vi "dv(SubVI).vi"(1 "Array in":dbl[][](array[numeric])) -> (0 "Array":dbl[][][](array[numeric]))   [LabVIEW 2021]
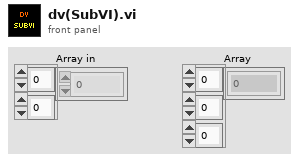
[diagram p1: front panel]
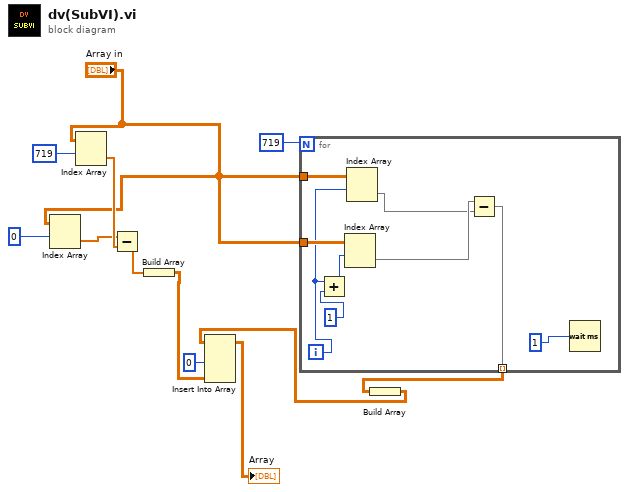
[diagram p0: block diagram]
diagram:
  n1 = Index Array "Index Array"(array="Array in", index (row)=0) -> (element=w7:dbl[])  [unwired: 1 in]
  n2 = Index Array(array="Array in", index (row)=719) -> (element=w8:dbl[])  [unwired: 1 in]
  n3 = Subtract(x=w7, y=w8) -> (x-y=w11:dbl[])
  n4 = Build Array(w11) -> (w12:dbl[][])
  n5 = for {
    N: 719 -> [_]
    tunnel: "Array in" -> [w20]
    tunnel: "Array in" -> [w16]
    tunnel: [w13] -> w4 mode=indexing
    i -> [w14]
    n6 = Add(x=w14, y=1) -> (x+y=w17:i32)
    n7 = Index Array "Index Array"(array=w20, index (row)=w17) -> (element=w19:dbl[])  [unwired: 1 in]
    n8 = Index Array "Index Array"(array=w16, index (row)=w14) -> (element=w15:dbl[])  [unwired: 1 in]
    n9 = Subtract(x=w19, y=w15) -> (x-y=w13:dbl[])
    n10 = Wait (ms)(milliseconds to wait=u32 1) -> ()  [unwired: 1 out]
  }
  n11 = Build Array(w4) -> (w3:dbl[][][])
  n12 = Insert Into Array(array=w3, index (dim 1)=0 ("disabled index (col)"), new element=w12) -> (→"Array":dbl[][][])  [unwired: 2 in]
